vi "Startup Engine.vi"(6 "LabVIEW Web Service":refnum<class "Web Service.lvclass">) -> ()   [LabVIEW 2014]
uses:
  <vilib>/wsapi/Web Service.lvclass
  Server Core/Coding Platform.lvlib
panel:
  # "Use the web service input terminal to call the VIs on the Service subpalette of the Web Services palette. Do not remove it from the connector pane unless you don't need access to the palette."
  # "Any additional terminals added to the connector pane of a startup VI will be ignored."
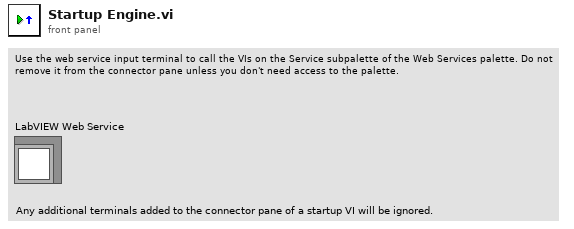
[diagram p1: front panel]
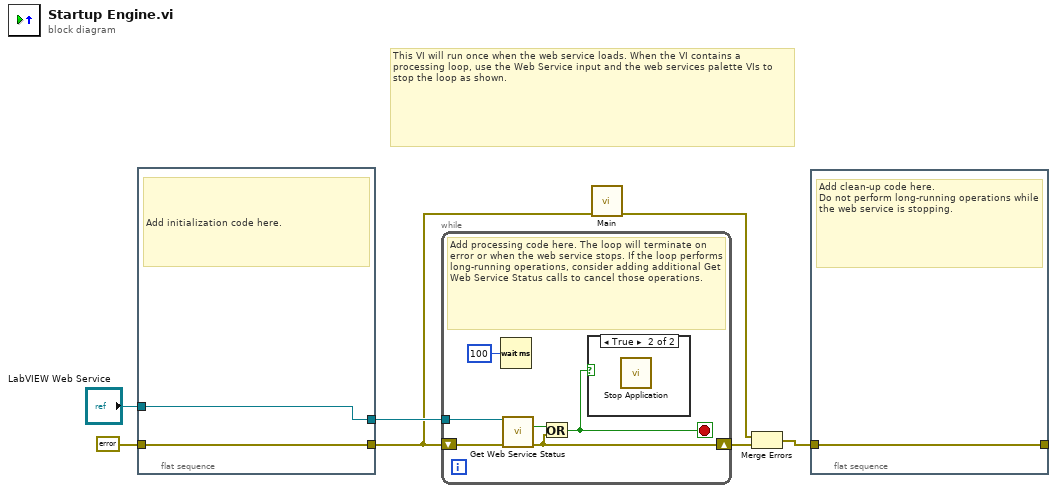
[diagram p0: block diagram]
diagram:
  # "This VI will run once when the web service loads. When the VI contains a processing loop, use the Web Service input and the web services palette VIs to stop the loop as shown."
  n1 = flat-sequence {
    tunnel: "LabVIEW Web Service" -> [w9]
    tunnel: [w9] -> w6
    tunnel: [w8] -> w3
    tunnel: errorcluster {"status"=FALSE, "code"=0, "source"=""} ("error constant") -> [w8]
    frame #0 {
      # "Add initialization code here."
    }
  }
  n2 = while {
    tunnel: w6 -> [w14]
    shift-right: [w13] -> w4
    shift-left: w3 -> [w11]
    stop <- w10 stop-if-true
    # "Add processing code here. The loop will terminate on error or when the web service stops. If the loop performs long-running operations, consider adding additional Get Web Service Status calls to cancel those operations."
    n3 = Wait (ms)(milliseconds to wait=u32 100) -> ()  [unwired: 1 out]
    n4 = call <vilib>:"Get Web Service Status.vi"("LabVIEW Web Service"=w14, "error in (no error)"=w11) -> ("service stopping?"=w15:bool, "error out"=w13:errorcluster)  [unwired: 11 in, 1 out]
    n5 = Or(x=w15, y=w13) -> (x .or. y?=w10:bool)
    n6 = case shown="True" w10 {
      frame False {
      }
      frame True {
        n7 = call "Stop Application.vi"() -> ()  [unwired: 15 in, 1 out]
      }
    }
  }
  n8 = call "Main.vi"("error in (no error)"=w3) -> ("error out"=w1:errorcluster)  [unwired: 14 in]
  n9 = Merge Errors(w1, w4) -> (w2:errorcluster)
  n10 = flat-sequence {
    tunnel: [w16] -> _
    tunnel: w2 -> [w16]
    frame #0 {
      # "Add clean-up code here.\nDo not perform long-running operations while the web service is stopping."
    }
  }
